vi "Host Page In Panel.vi"(8 "error in (no error)":errorcluster, 9 "Node Ptr":T1 format="%.0x", 10 "vi path":path, 11 "SubPanel in":refnum<vi>) -> (0 "error out":errorcluster)   [LabVIEW 2015, in "Engine Simulation Toolkit System Explorer.lvlib"]
uses:
  Engine Simulation Toolkit System Explorer.lvlib
  <vilib>/NI Veristand/Custom Device API/Custom Device Item Ref.ctl
  <vilib>/NI Veristand/Custom Device API/Custom Device API.lvlib
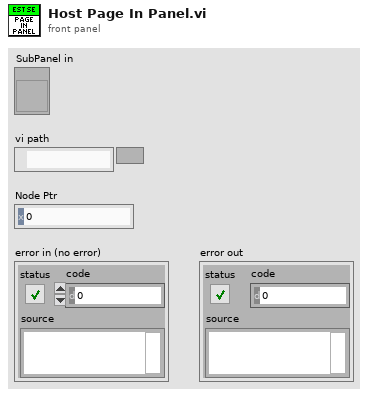
[diagram p1: front panel]
types:
  T1 = typedef "Custom Device API.lvlib/Custom Device Item Ref.ctl" = u64
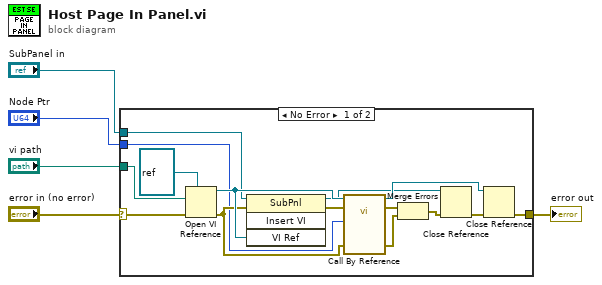
[diagram p0: block diagram]
diagram:
  n1 = case shown="No Error" "error in (no error)" {
    selector: "error in (no error)" -> [w8 w21]
    tunnel: [w14 w21] -> w5
    tunnel: "vi path" -> [w13 _]
    tunnel: "SubPanel in" -> [w9 _]
    tunnel: "Node Ptr" -> [w6 _]
    frame No Error {
      n2 = Open VI Reference(type specifier VI Refnum (for type only)=refnum<vi> refnum, vi path=w13, error in (no error)=w8) -> (vi reference=w16:refnum<vi>, error out=w10:errorcluster)  [unwired: 3 in]
      n3 = invoke on="Invoke Node" class="SubPnl" method="Insert VI"(reference=w9, error in=w10, "VI Ref"=w16) -> (reference out=w11:refnum<vi>, error out=w20:errorcluster)  [unwired: 1 in, 2 out]
      n4 = call-by-ref "?"(reference=w16, error in=w20, 8:"error in (no error)"=w10, "Node Ptr"=w6) -> (reference out=w17:refnum<vi>, error out=w19:errorcluster, 0:"error out"=w18:errorcluster)  [unwired: 9 in]
      n5 = Merge Errors(w19, w18) -> (w15:errorcluster)
      n6 = Close Reference(reference=w11, error in (no error)=w15) -> (error out=w7:errorcluster)
      n7 = Close Reference(reference=w17, error in (no error)=w7) -> (error out=w14:errorcluster)
    }
    frame Error {
    }
  }
  "error out" <- w5
